vi "ws key accept process.vi"() -> ()   [LabVIEW 2016]
uses:
  http/websocket/websocket core.lvlib
panel:
  out "x = y?":bool
  out "string out (base64-encoded)":string
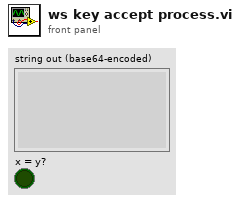
[diagram p1: front panel]
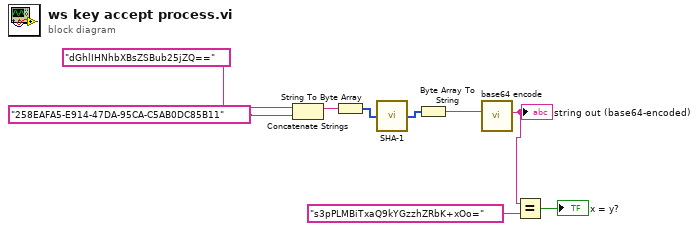
[diagram p0: block diagram]
diagram:
  n1 = Concatenate Strings("dGhlIHNhbXBsZSBub25jZQ==" ("string"), "258EAFA5-E914-47DA-95CA-C5AB0DC85B11") -> (w8:string)
  n2 = String To Byte Array(string=w8) -> (unsigned byte array=w7:u8[])
  n3 = call "SHA-1.vi"("Data"=w7) -> ("message-digest"=w6:u8[])
  n4 = Byte Array To String(unsigned byte array=w6) -> (string=w5:string)
  n5 = call "base64 encode.vi"("string in (not encoded)"=w5) -> ("string out (base64-encoded)"=w3:string)  [unwired: 10 in]
  "string out (base64-encoded)" <- w3
  n6 = Equal?(x=w3, y="s3pPLMBiTxaQ9kYGzzhZRbK+xOo=") -> (x = y?=→"x = y?":bool)
